vi "SCCSup Dialog_GenMCLB_ShowHScroll.vi"(11 "Multicolumn Listbox":refnum<vi>) -> (1 "pixels from edge":u32, 2 "numColumns":i32, 3 "show HScrollbar?":bool)   [LabVIEW 2017]
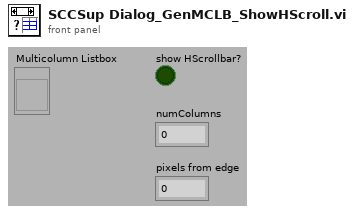
[diagram p1: front panel]
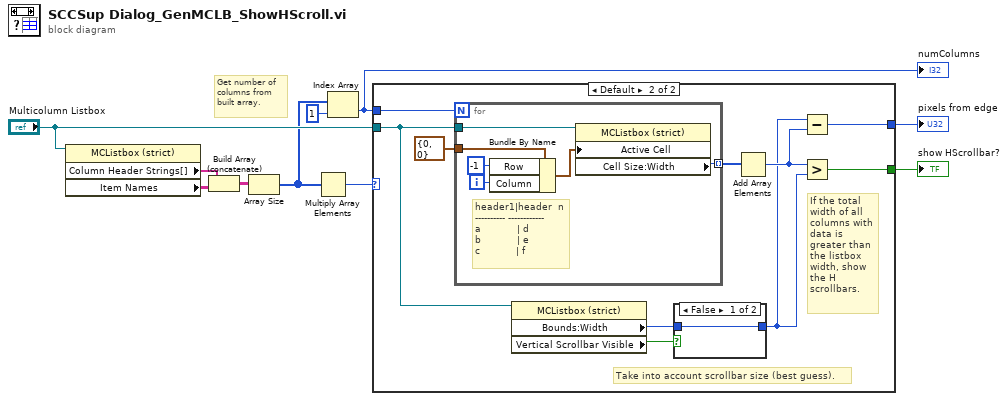
[diagram p0: block diagram]
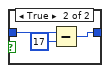
[diagram p3: hidden frame]
diagram:
  # "Get number of columns from built array."
  n1 = property on="Property Node" class="MCListbox (strict)"(reference="Multicolumn Listbox") -> ("Column Header Strings[]"=w7:string[], "Item Names"=w9:string[][])  [unwired: 1 in, 2 out]
  n2 = Build Array (concatenate)(w7, w9) -> (w8:string[][])
  n3 = Array Size(array=w8) -> (size(s)=w2:i32[])
  n4 = Multiply Array Elements(1:w2) -> (0:w6:i32)
  n5 = Index Array(array=w2, index=1) -> (element=w1:i32)
  "numColumns" <- w1
  n6 = case shown="Default" w6 {
    tunnel: "Multicolumn Listbox" -> [_ w18]
    tunnel: [_ w17] -> w5
    tunnel: [_ w15] -> w4
    tunnel: w1 -> [_ w14]
    frame 0 {
      # "Don't do anything if no data in listbox."
    }
    frame Default {
      # "Take into account scrollbar size (best guess)."
      # "If the total width of all columns with data is greater than the listbox width, show the H scrollbars."
      n7 = for {
        N: w14 -> [_]
        tunnel: cluster{"Row":i32, "Column":i32} {"Row"=0, "Column"=0} ("Active Cell") -> [w27]
        tunnel: [w30] -> w19 mode=indexing
        tunnel: w18 -> [w29]
        i -> [w25]
        # "header1|header  n\n---------- ------------\na            | d\nb            | e\nc            | f"
        n8 = Bundle By Name(cluster=w27, "Row"=-1, "Column"=w25) -> (w26:cluster{"Row":i32, "Column":i32})
        n9 = property on="Property Node" class="MCListbox (strict)"(reference=w29, "Active Cell"=w26) -> ("Cell Size:Width"=w30:u32)  [unwired: 1 in, 2 out]
      }
      n10 = property on="Property Node" class="MCListbox (strict)"(reference=w18) -> ("Bounds:Width"=w12:u32, "Vertical Scrollbar Visible"=w13:bool)  [unwired: 1 in, 2 out]
      n11 = case shown="False" w13 {
        tunnel: w12 -> [w21 w24]
        tunnel: [w21 w22] -> w11
        frame False {
        }
        frame True {
          n12 = Subtract(x=w24, y=u32 17) -> (x-y=w22:u32)
        }
      }
      n13 = Add Array Elements(numeric array=w19) -> (sum=w16:u32)
      n14 = Subtract(x=w11, y=w16) -> (x-y=w15:u32)
      n15 = Greater?(x=w16, y=w11) -> (0:w17:bool)
    }
  }
  "show HScrollbar?" <- w5
  "pixels from edge" <- w4
